vi "Rpt _Get _HWShip Data.vi"(0 "Traceability 引用句柄":refnum<k24>, 1 "DateTo":string, 2 ".NET:System.Data.DataSet":T1={"CaseSensitive"=FALSE, "Container"=refnum, "DataSetName"="", "DefaultViewManager"=refnum, "DesignMode"=FALSE, "EnforceConstraints"=FALSE, "ExtendedProperties"=refnum, "HasErrors"=FALSE, "IsInitialized"=FALSE, "Locale"=refnum, "Namespace"="", "Prefix"="", "Relations"=refnum, "RemotingFormat"=0, "SchemaSerializationMode"=1, "Site"=refnum, "Tables"=refnum} {"SchemaSerializationMode" items=["IncludeSchema"=1, "ExcludeSchema"=2]; "RemotingFormat" items=["Xml", "Binary"]}, 3 "PackingDTTo":string, 5 "Model":string, 7 "DateCode":string, 9 "DateFrom":string, 11 "error in (no error)":errorcluster caption="错误输入（无错误）", 12 "HD":string, 13 "PackingDTFrm":string) -> (4 "Traceability 引用句柄输出":refnum<k24>, 6 ".NET:System.Data.DataSet":T1={"CaseSensitive"=FALSE, "Container"=refnum, "DataSetName"="", "DefaultViewManager"=refnum, "DesignMode"=FALSE, "EnforceConstraints"=FALSE, "ExtendedProperties"=refnum, "HasErrors"=FALSE, "IsInitialized"=FALSE, "Locale"=refnum, "Namespace"="", "Prefix"="", "Relations"=refnum, "RemotingFormat"=0, "SchemaSerializationMode"=1, "Site"=refnum, "Tables"=refnum} {"SchemaSerializationMode" items=["IncludeSchema"=1, "ExcludeSchema"=2]; "RemotingFormat" items=["Xml", "Binary"]}, 15 "error out":errorcluster caption="错误输出")   [LabVIEW 2014, in "Traceability.lvlib"]
uses:
  Traceability.lvlib
  Traceability.dll
  System.Data
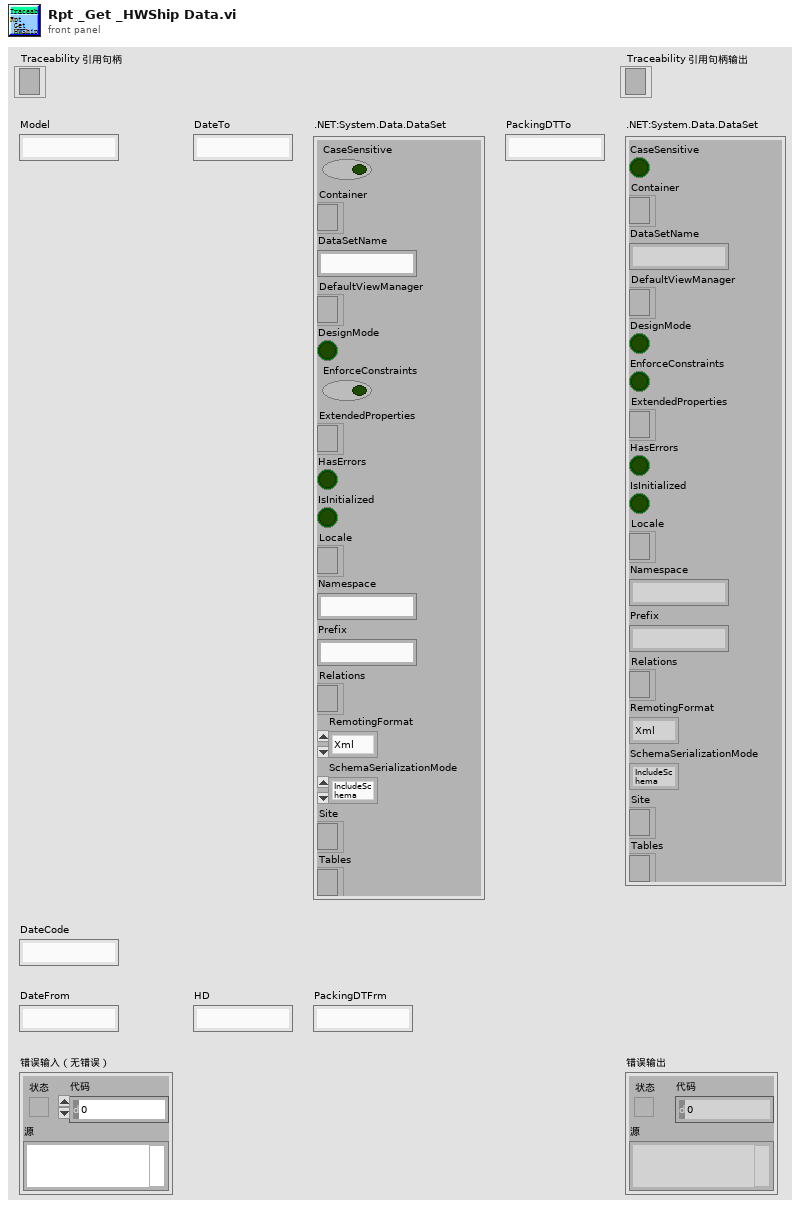
[diagram p1: front panel]
types:
  T1 = cluster{"CaseSensitive":bool, "Container":refnum<k24>, "DataSetName":string, "DefaultViewManager":refnum<k24>, "DesignMode":bool, "EnforceConstraints":bool, "ExtendedProperties":refnum<k24>, "HasErrors":bool, "IsInitialized":bool, "Locale":refnum<k24>, "Namespace":string, "Prefix":string, "Relations":refnum<k24>, "RemotingFormat":i32, "SchemaSerializationMode":i32, "Site":refnum<k24>, "Tables":refnum<k24>}
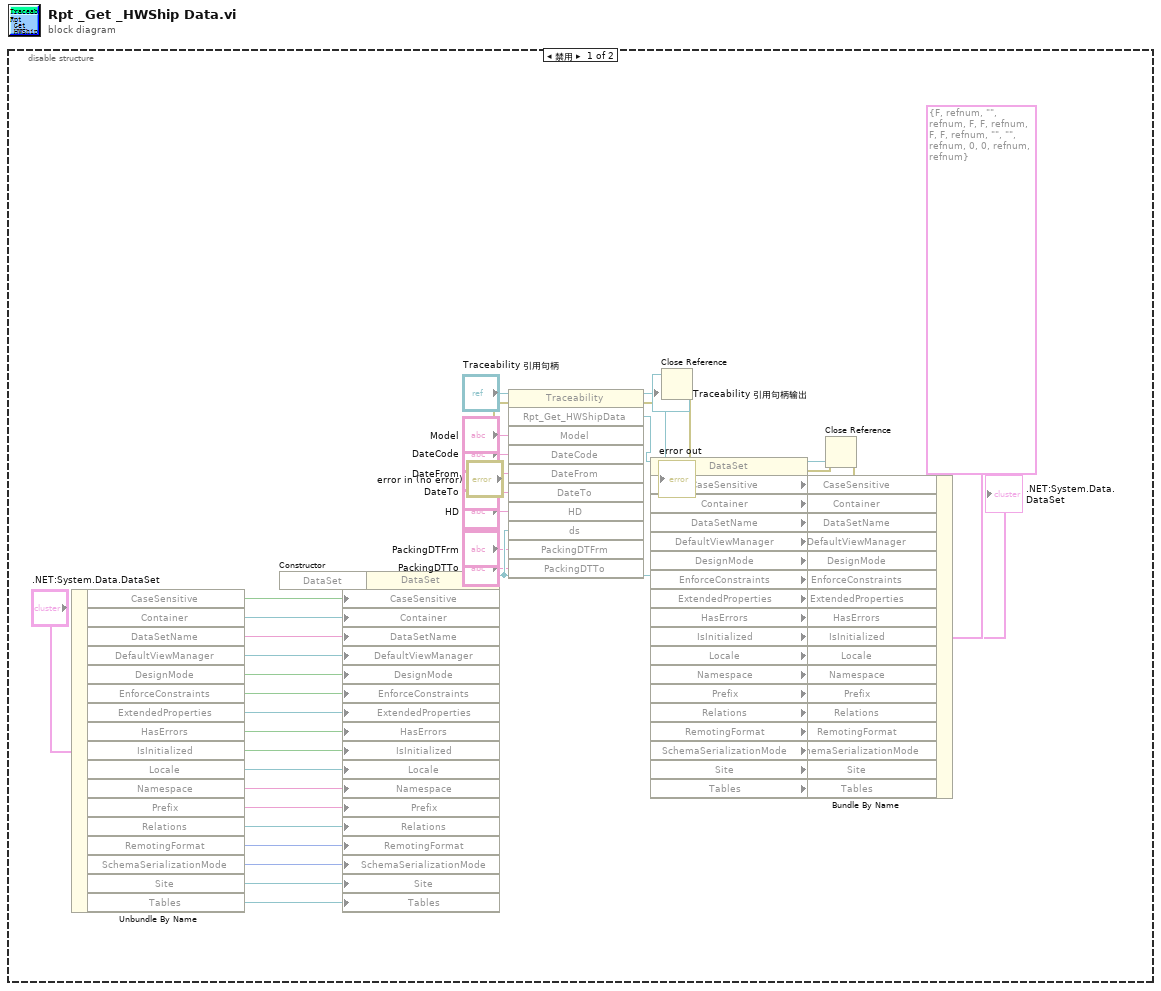
[diagram p0: block diagram]
diagram:
  n1 = disable-structure shown="禁用" {
    frame Disabled {
      n2 = Unbundle By Name(".NET:System.Data.DataSet") -> ("CaseSensitive"=w26:bool, "Container"=w25:refnum<k24>, "DataSetName"=w24:string, "DefaultViewManager"=w23:refnum<k24>, "DesignMode"=w22:bool, "EnforceConstraints"=w21:bool, "ExtendedProperties"=w20:refnum<k24>, "HasErrors"=w19:bool, "IsInitialized"=w18:bool, "Locale"=w17:refnum<k24>, "Namespace"=w16:string, "Prefix"=w15:string, "Relations"=w14:refnum<k24>, "RemotingFormat"=w13:i32, "SchemaSerializationMode"=w12:i32, "Site"=w11:refnum<k24>, "Tables"=w10:refnum<k24>)
      n3 = constructor class="DataSet"(error in="error in (no error)") -> (reference out=w30:refnum<k24>, error out=w29:errorcluster)  [unwired: 2 in, 1 out]
      n4 = property class="DataSet"(reference=w30, error in=w29, "CaseSensitive"=w26, "Container"=w25, "DataSetName"=w24, "DefaultViewManager"=w23, "DesignMode"=w22, "EnforceConstraints"=w21, "ExtendedProperties"=w20, "HasErrors"=w19, "IsInitialized"=w18, "Locale"=w17, "Namespace"=w16, "Prefix"=w15, "Relations"=w14, "RemotingFormat"=w13, "SchemaSerializationMode"=w12, "Site"=w11, "Tables"=w10) -> (reference out=w28:refnum<k24>, error out=w6:errorcluster)
      n5 = invoke class="Traceability" method="Rpt_Get_HWShipData"(reference="Traceability 引用句柄", error in=w6, "Model"="Model", "DateCode"="DateCode", "DateFrom"="DateFrom", "DateTo"="DateTo", "HD"="HD", "ds"=w28, "PackingDTFrm"="PackingDTFrm", "PackingDTTo"="PackingDTTo") -> (reference out=→"Traceability 引用句柄输出":refnum<k24>, error out=w5:errorcluster, "Rpt_Get_HWShipData"=w55:refnum<k24>)  [unwired: 1 in, 8 out]
      n6 = Close Reference(reference=w28, error in (no error)=w5) -> (error out=w4:errorcluster)
      n7 = property class="DataSet"(reference=w55, error in=w4) -> (reference out=w3:refnum<k24>, error out=w2:errorcluster, "CaseSensitive"=w52:bool, "Container"=w51:refnum<k24>, "DataSetName"=w50:string, "DefaultViewManager"=w49:refnum<k24>, "DesignMode"=w48:bool, "EnforceConstraints"=w47:bool, "ExtendedProperties"=w46:refnum<k24>, "HasErrors"=w45:bool, "IsInitialized"=w44:bool, "Locale"=w43:refnum<k24>, "Namespace"=w42:string, "Prefix"=w41:string, "Relations"=w40:refnum<k24>, "RemotingFormat"=w39:i32, "SchemaSerializationMode"=w38:i32, "Site"=w37:refnum<k24>, "Tables"=w36:refnum<k24>)
      n8 = Bundle By Name(cluster=T1 {"CaseSensitive"=FALSE, "Container"=refnum, "DataSetName"="", "DefaultViewManager"=refnum, "DesignMode"=FALSE, "EnforceConstraints"=FALSE, "ExtendedProperties"=refnum, "HasErrors"=FALSE, "IsInitialized"=FALSE, "Locale"=refnum, "Namespace"="", "Prefix"="", "Relations"=refnum, "RemotingFormat"=0, "SchemaSerializationMode"=0, "Site"=refnum, "Tables"=refnum} (".NET:System.Data.DataSet"), "CaseSensitive"=w52, "Container"=w51, "DataSetName"=w50, "DefaultViewManager"=w49, "DesignMode"=w48, "EnforceConstraints"=w47, "ExtendedProperties"=w46, "HasErrors"=w45, "IsInitialized"=w44, "Locale"=w43, "Namespace"=w42, "Prefix"=w41, "Relations"=w40, "RemotingFormat"=w39, "SchemaSerializationMode"=w38, "Site"=w37, "Tables"=w36) -> (→".NET:System.Data.DataSet":T1)
      n9 = Close Reference(reference=w3, error in (no error)=w2) -> (error out=→"error out":errorcluster)
    }
    frame Enabled {
    }
  }
